vi "Get Pot Home Values.vi"() -> (0 "Front Left":dbl, 1 "Rear Left":dbl, 2 "Front Right":dbl, 3 "Rear Right":dbl)   [LabVIEW 2012]
uses:
  Globals/Pot Home Values.vi
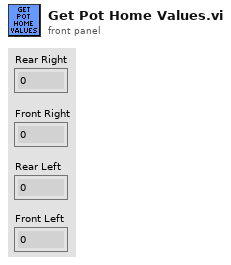
[diagram p1: front panel]
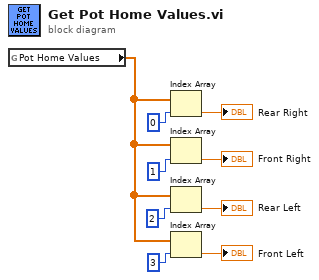
[diagram p0: block diagram]
diagram:
  n1 = global read "Pot Home Values.vi" "Pot Home Values"() -> (w5:dbl[])
  n2 = Index Array(array=w5, index=0) -> (element=→"Rear Right":dbl)
  n3 = Index Array(array=w5, index=1) -> (element=→"Front Right":dbl)
  n4 = Index Array(array=w5, index=2) -> (element=→"Rear Left":dbl)
  n5 = Index Array(array=w5, index=3) -> (element=→"Front Left":dbl)
